vi "Write Person.vi"(10 "Person":T1 {"Birth Date" format="%<%Y/%b/%d>T"}, 11 "People Wrapper in":refnum<class "People By Month Wrapper.lvclass">) -> (3 "People Wrapper out":refnum<class "People By Month Wrapper.lvclass">)   [LabVIEW 2023, in "People By Month Wrapper.lvclass"]
uses:
  People By Month Wrapper.lvclass
  Person Information.ctl
  People By Month Wrapper.lvclass/People By Month Wrapper.ctl
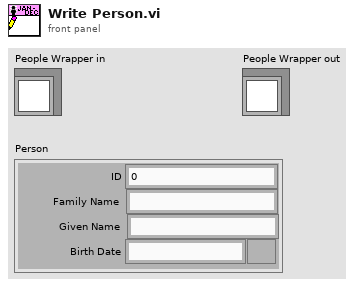
[diagram p1: front panel]
types:
  T1 = typedef "Person Information.ctl" = cluster{"ID":u32, "Family Name":string, "Given Name":string, "Birth Date":timestamp}
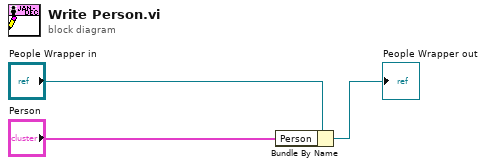
[diagram p0: block diagram]
diagram:
  n1 = Bundle By Name(cluster="People Wrapper in", "Person"="Person") -> (→"People Wrapper out":refnum<class "People By Month Wrapper.lvclass">)
